vi "switchOn.vi"(8 "error in (no error)":errorcluster, 11 "AndorIKonTempController in":refnum<class "AndorIKonTempController.lvclass">) -> (0 "error out":errorcluster, 3 "AndorIKonTempController out":refnum<class "AndorIKonTempController.lvclass">)   [LabVIEW 2009, in "Hardware.lvlib" / "Channels.lvlib" / "AndorIKonTempController.lvclass"]
uses:
  AndorIKonTempController.lvclass
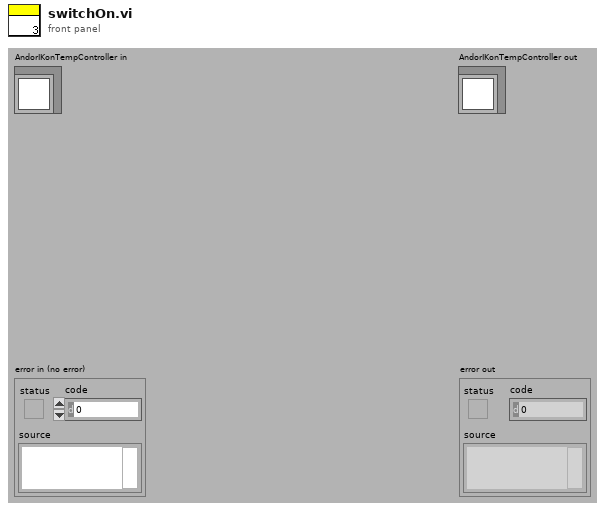
[diagram p1: front panel]
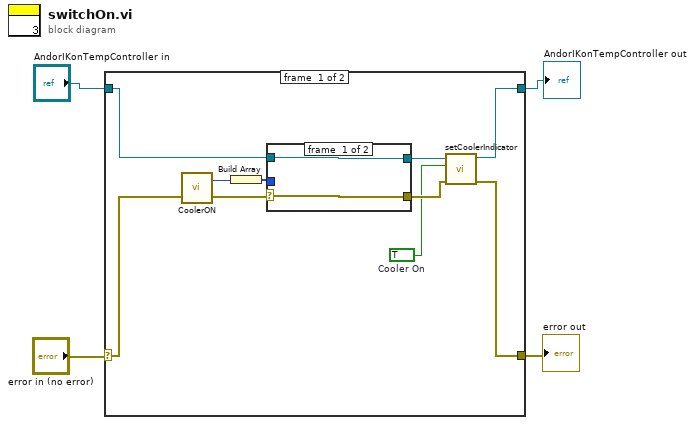
[diagram p0: block diagram]
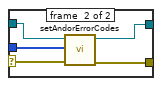
[diagram p2: hidden frame]
diagram:
  n1 = case shown="No Error" "error in (no error)" {
    selector: "error in (no error)" -> [w11 w22]
    tunnel: "AndorIKonTempController in" -> [w10 w23]
    tunnel: [w6 w23] -> w2
    tunnel: [w7 w22] -> w1
    frame #0 {
      w5 = TRUE  # Cooler On
      n2 = call <userlib>:"CoolerON.vi"("error in (no error)"=w11) -> ("error out"=w12:errorcluster, "DLL error code"=w13:u32)  [unwired: 1 in]
      n3 = Build Array(w13) -> (w14:u32[])
      n4 = case shown="Error" w12 {
        selector: w12 -> [w16 w19]
        tunnel: [w16 w18] -> w8
        tunnel: w14 -> [_ w21]
        tunnel: w10 -> [w15 w20]
        tunnel: [w15 w17] -> w9
        frame #0 {
        }
        frame #1 {
          n5 = call-dynamic "setAndorErrorCodes.vi"("error in (no error)"=w19, "Andor Error Codes"=w21, "AndorIKonTempController.lvclass in"=w20) -> ("error out"=w18:errorcluster, "AndorIKonTempController.lvclass out"=w17:refnum<class "AndorIKonTempController.lvclass">)  [unwired: 7 in]
        }
      }
      n6 = call-dynamic "setCoolerIndicator.vi"("error in (no error)"=w8, "Cooler"=w5, "CameraTempController.lvclass in"=w9) -> ("error out"=w7:errorcluster, "CameraTempController.lvclass out"=w6:refnum<class "AndorIKonTempController.lvclass">)  [unwired: 7 in]
    }
    frame #1 {
    }
  }
  "error out" <- w1
  "AndorIKonTempController out" <- w2
